vi "Limit range based on sensors.vi"(4 "Position":dbl, 6 "Position Max":dbl, 7 "min speed":dbl=-0.1 format="%#_13g", 10 "output low":dbl, 11 "output high":dbl) -> (2 "output low":dbl, 3 "output high":dbl)   [LabVIEW 2018]
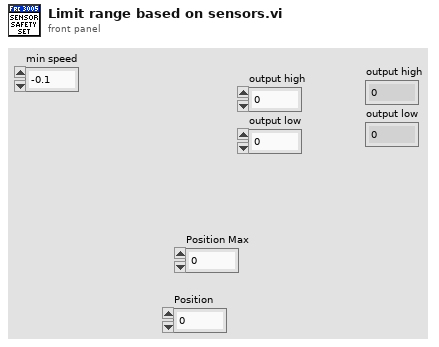
[diagram p1: front panel]
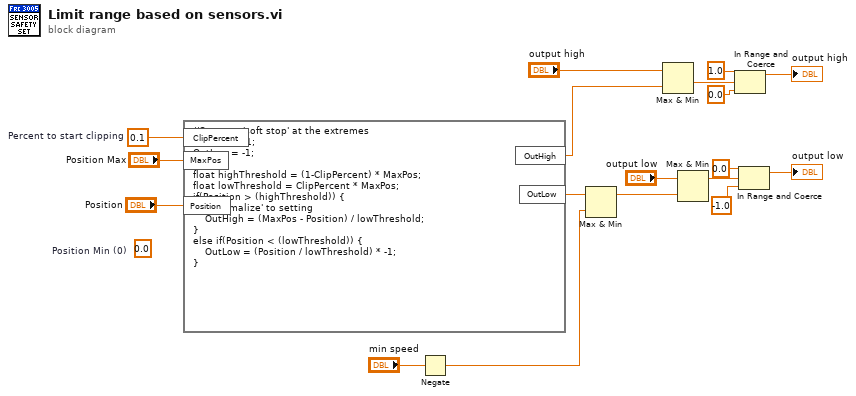
[diagram p0: block diagram]
diagram:
  w17 = 0.1  # Percent to start clipping
  (unwired) 0.0  # Position Min (0)
  n1 = formula code="//Create a 'soft stop' at the extremes\nOutHigh = 1;\nOutLow = -1;\n\nfloat highThreshold = (1-ClipPercent) * MaxPos;\nfloat lowThreshold = ClipPercent * MaxPos;\nif(Position > (highThreshold)) {\n    //'normalize' to setting\n    OutHigh = (MaxPos - Position) / lowThreshold;\n}\nelse if(Position < (lowThreshold)) {\n    OutLow = (Position / lowThreshold) * -1;\n}"("MaxPos"="Position Max", "ClipPercent"=w17, "Position"="Position") -> ("OutHigh"=w13:dbl, "OutLow"=w14:dbl)
  n2 = Negate(x="min speed") -> (-x=w5:dbl)
  n3 = Max & Min(x=w14, y=w5) -> (max(x,y)=w10:dbl)  [unwired: 1 out]
  n4 = Max & Min(x="output high", y=w13) -> (min(x,y)=w12:dbl)  [unwired: 1 out]
  n5 = Max & Min(x="output low", y=w10) -> (max(x,y)=w11:dbl)  [unwired: 1 out]
  n6 = In Range and Coerce(upper limit=1.0, x=w12, lower limit=0.0) -> (coerced(x)=→"output high":dbl)  [unwired: 1 out]
  n7 = In Range and Coerce(upper limit=0.0, x=w11, lower limit=-1.0) -> (coerced(x)=→"output low":dbl)  [unwired: 1 out]
